vi "Edgertronic-configure.vi"(0 "URL":string, 1 "GET Command":string="/configure_camera", 2 "Post":string, 3 "error in (no error)":errorcluster) -> (6 "Saved Settings:":T1={"Requested Genlock "="20140911165611", "Min Frame Clocks "="20140911165611", "Is Seq Clk Freq "="20140911165611", "Pretrigger Frames "="20140911165611", "Duration "="20140911165611", "Overclock "="20140911165611", "Requested Horizontal "="20140911165611", "Frames "="20140911165611", "Requested Pretrigger "="20140911165611", "Words per Frame "="20140911165611", "Buffer End "="20140911165611", "Clocks per Frame  "="20140911165611", "Requested Duration "="20140911165611", "Pretrigger "="20140911165611", "Post-trigger Frames "="20140911165611", "Vertical "="20140911165611", "Requested Vertical "="20140911165611", "Reqested Frame Rate "="20140911165611", "Frame Rate "="20140911165611", "Horizontal "="20140911165611", "Clocks per Exposure "="20140911165611", "Digital Gain "="20140911165611", "Exposure "="20140911165611", "Genlock "="20140911165611", "Analog Gain "="20140911165611", "Subsample "="20140911165611", "Requested Exposure "="20140911165611", "Iso "="20140911165611", "Requested Overclock "="20140911165611", "Requested Subsample "="20140911165611", "Requested Iso"="20140911165611", "Multishot"="20140911165611", "Requested Multishot"="20140911165611", "Monochrome"="20140911165611", "Requested mono"="20140911165611", "FPGA Temp"="20140911165611", "Is Temp"="20140911165611", "Posttrigger Duration"="20140911165611", "Pretrigger Duration"="20140911165611", "dacvrefadc"="20140911165611"}, 7 "error out":errorcluster)   [LabVIEW 2015]
panel:
  out "Reply":string="{\"requested_horizontal\": \"733\", \"requested_vertical\": \"831\", \"requested_frame_rate\": \"1000.00\", \"requested_exposure\": \"0.002000\", \"requested_duration\": \"1.00\", \"requested_pretrigger\": \"50\", \"requested_iso\": \"500\", \"requested_subsample\": \"0\", \"requested_genlock\": \"0\", \"requested_overclock\": \"0\", \"requested_force_mono\": \"0\"}"
  out "Connection Information":string="HTTP/1.1 200 OK\r\nAccess-Control-Allow-Origin: *\r\nContent-Type: text/html; charset=utf-8\r\nContent-Length: 899\r\nDate: Fri, 01 Jul 2016 15:58:52 GMT\r\nServer: lighttpd/1.4.11 (edgertonic slow motion camera)\r\n\r\n"
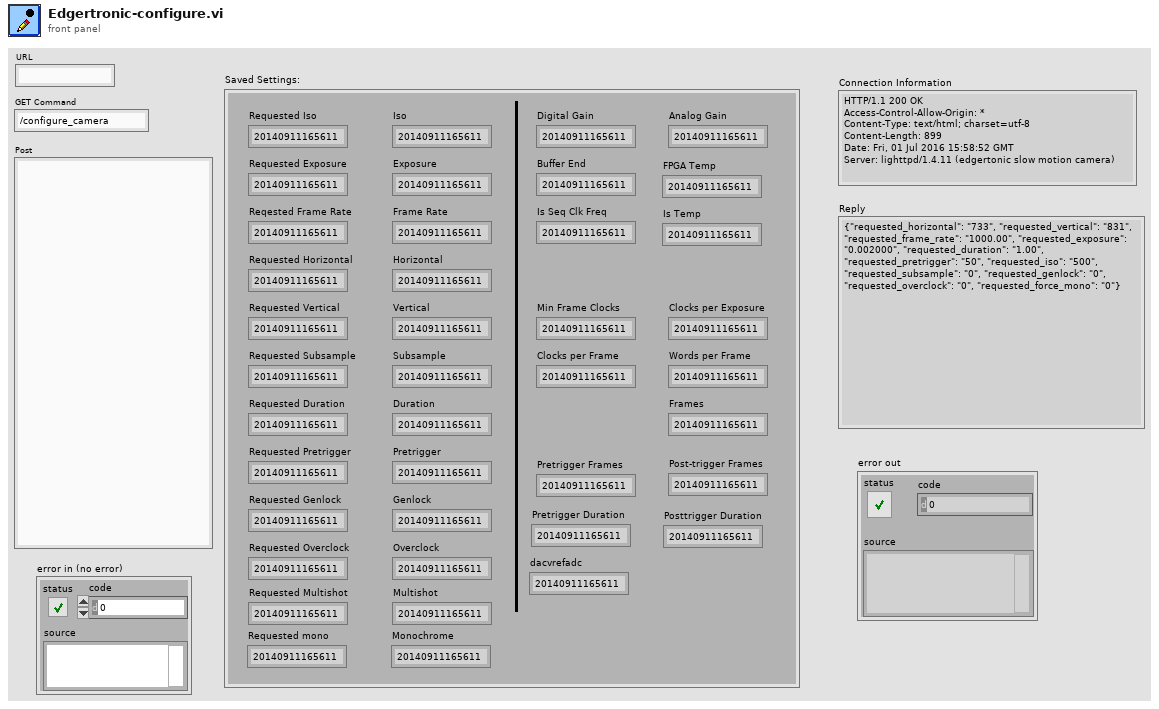
[diagram p1: front panel]
types:
  T1 = cluster{"Requested Genlock ":string, "Min Frame Clocks ":string, "Is Seq Clk Freq ":string, "Pretrigger Frames ":string, "Duration ":string, "Overclock ":string, "Requested Horizontal ":string, "Frames ":string, "Requested Pretrigger ":string, "Words per Frame ":string, "Buffer End ":string, "Clocks per Frame  ":string, "Requested Duration ":string, "Pretrigger ":string, "Post-trigger Frames ":string, "Vertical ":string, "Requested Vertical ":string, "Reqested Frame Rate ":string, "Frame Rate ":string, "Horizontal ":string, "Clocks per Exposure ":string, "Digital Gain ":string, "Exposure ":string, "Genlock ":string, "Analog Gain ":string, "Subsample ":string, "Requested Exposure ":string, "Iso ":string, "Requested Overclock ":string, "Requested Subsample ":string, "Requested Iso":string, "Multishot":string, "Requested Multishot":string, "Monochrome":string, "Requested mono":string, "FPGA Temp":string, "Is Temp":string, "Posttrigger Duration":string, "Pretrigger Duration":string, "dacvrefadc":string}
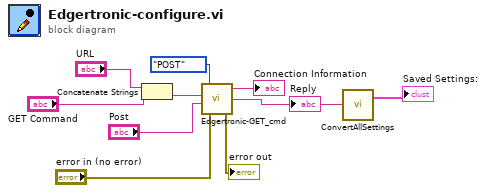
[diagram p0: block diagram]
diagram:
  n1 = Concatenate Strings("URL", "GET Command") -> (w8:string)
  n2 = call "Edgertronic-GET_cmd.vi"("error in (no error)"="error in (no error)", "Posted Content"="Post", "URL"=w8, "Type"=enum16{"GET", "POST"}."POST") -> ("error out"=→"error out":errorcluster, "data"=w2:string, "Connection Info"=→"Connection Information":string)
  "Reply" <- w2
  n3 = call "ConvertAllSettings.vi"("data"=w2) -> ("Saved Settings:"=→"Saved Settings:":T1)  [unwired: 2 in]
